vi "EsportaLog.vi"(11 "TABELLA LOG":refnum<vi>) -> ()   [LabVIEW 2019]
uses:
  <vilib>/Utility/NIReport.llb/Report Type.ctl
  <vilib>/addons/_office/excel.llb/Excel Easy Table (str).vi
  <vilib>/Utility/NIReport.llb/NI_report.lvclass
  <vilib>/Utility/NIReport.llb/Excel/NI_Excel.lvclass
  <vilib>/addons/_office/NI_ReportGenerationToolkit.lvlib
  <vilib>/Utility/NIReport.llb/NI_ReportGenerationCore.lvlib
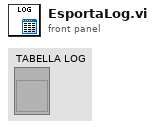
[diagram p1: front panel]
types:
  T1 = enum16{"maximized", "minimized", "normal", "no change"}
  T2 = typedef "NI_ReportGenerationCore.lvlib/Report Type.ctl" = enum16{"HTML", "Word", "Excel"}
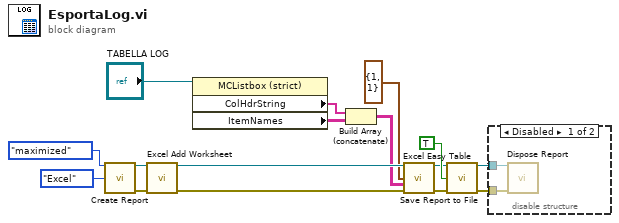
[diagram p0: block diagram]
diagram:
  n1 = call <vilib>:"Create Report.vi"("window state (normal)"=T1."maximized", "report type"=Report_Type."Excel") -> ("report out"=w2:refnum<class "NI_report.lvclass">, "error out"=w1:errorcluster)  [unwired: 12 in]
  n2 = call <vilib>:"Excel Add Worksheet.vi"("report in"=w2, "error in (no error)"=w1) -> ("report out"=w16:refnum<class "NI_report.lvclass">, "error out"=w15:errorcluster)  [unwired: 12 in]
  n3 = property class="MCListbox (strict)"(reference="TABELLA LOG") -> ("ColHdrString"=w12:string[], "ItemNames"=w11:string[][])  [unwired: 1 in, 2 out]
  n4 = Build Array (concatenate)(w12, w11) -> (w10:string[][])
  n5 = call-poly <vilib>:"Excel Easy Table.vi"("report in"=w16, "start (0, 0)"=cluster{"row":i32, "column":i32} {"row"=1, "column"=1}, "text data"=w10, "error in (no error)"=w15) -> ("report out"=w8:refnum<class "NI_report.lvclass">, "error out"=w7:errorcluster)  [unwired: 7 in, 3 out]
  n6 = call-dynamic "Save Report to File.vi"("report in"=w8, "prompt to replace? (F)"=TRUE, "error in (no error)"=w7) -> ("report out"=w6:refnum<class "NI_report.lvclass">, "error out"=w5:errorcluster)  [unwired: 11 in]
  n7 = disable-structure shown="Disabled" {
    disable-tunnel: w6 -> [w18 _]
    disable-tunnel: w5 -> [w17 _]
    frame Disabled {
      n8 = call-dynamic "Dispose Report.vi"("report in"=w18, "error in (no error)"=w17) -> ()  [unwired: 13 in, 1 out]
    }
    frame Enabled {
    }
  }
